vi "FTW-TestExecutive-Core_Process.vi"(0 "FTW Actor Instance Configuration":string="{\n  \"Identity\": \"FTW Test Executive\",\n  \"InboxAddress\": \"inproc://ftwTestExec\",\n  \"LoggerAddress\": \"\",\n  \"Connections\": {},\n  \"Publishers\": {\n    \"TestExecStatus\": \"inproc://testExecStatus\"\n  },\n  \"Subscriptions\": {},\n  \"Step Name Dictionary\": {},\n  \"Refresh Period\": 0.1\n}", 11 "ErrorIn":errorcluster) -> (15 "Error":errorcluster)   [LabVIEW 2015, in "FTW-TestExecutive-Core.lvclass"]
uses:
  FTW-TestExecutive-Core.lvclass
  source/actor/Instance/FTW-ActorInstance.lvclass
  source/actor/Message/Request/FTW-Message-IncomingRequest.lvclass
  source/actor/Message/Base/FTW-Message.lvclass
  source/actor/Instance-Extended/FTW-ActorExtended.lvclass
  Test Steps/Wait/FTW-TestStep-Wait-Core_Step.vi
  Test Steps/Wait/FTW-TestStep-Wait-Core.lvclass
  FTW-TestExecutive-Core_State.ctl
  FTW-TestExecutive-Core_Step_State.ctl
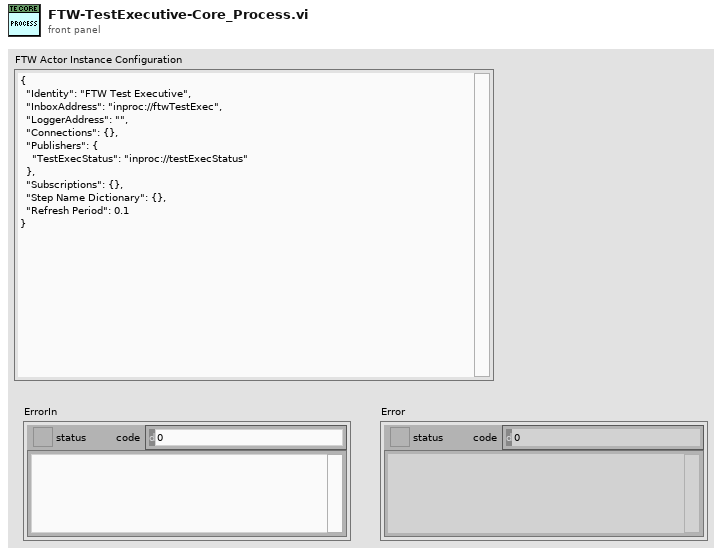
[diagram p1: front panel]
types:
  T1 = cluster{"Incoming Requests":refnum<event-registration>, "Local Messages":refnum<event-registration>, "Subscriber Registration":refnum<event-registration>}
  T2 = typedef "FTW-TestExecutive-Core.lvclass/FTW-TestExecutive-Core_Step_State.ctl" = enum8{"None", "Failed", "Passed", "Timed out", "Aborted"}
  T3 = typedef "FTW-TestExecutive-Core.lvclass/FTW-TestExecutive-Core_State.ctl" = enum8{"Unloaded", "Loaded", "Executing", "Paused"}
  T4 = typedef "FTW-TestExecutive_Step.ctl" = cluster{"Name":string, "Type":string, "Path":string, "Config":string, "Elapsed Time":dbl, "Passed":bool}
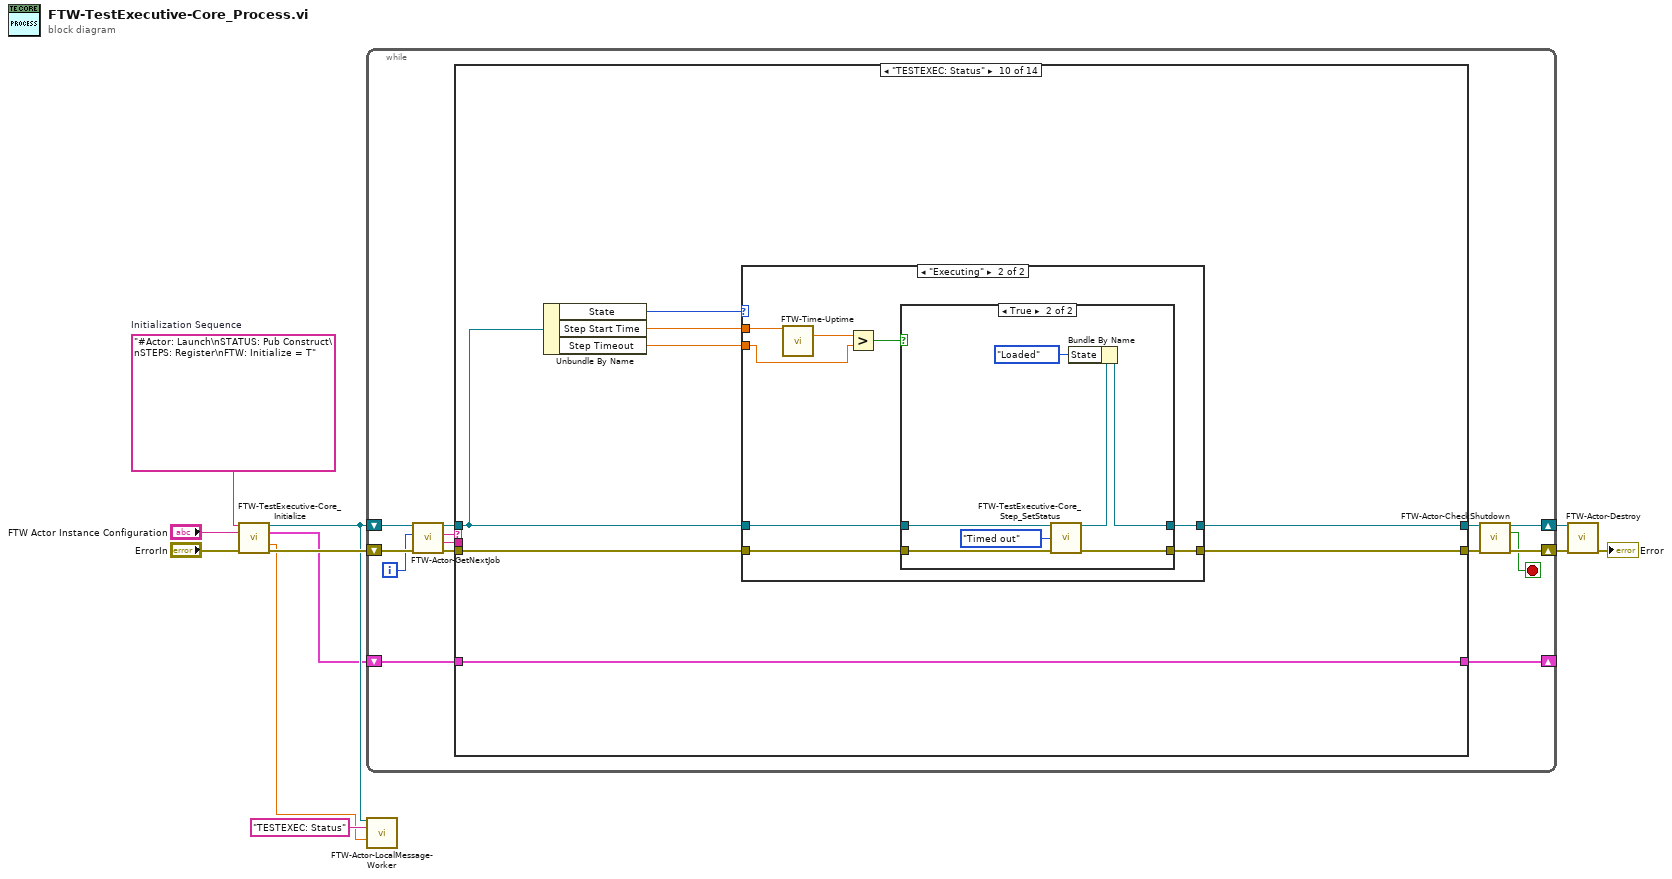
[diagram p0: block diagram]
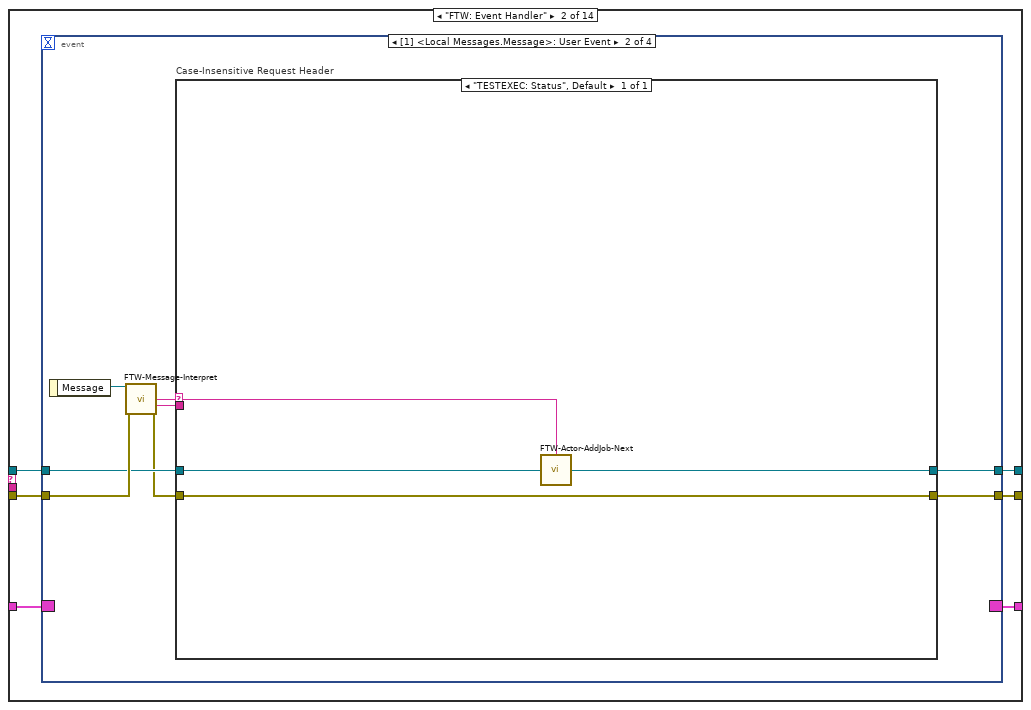
[diagram p3: hidden frame]
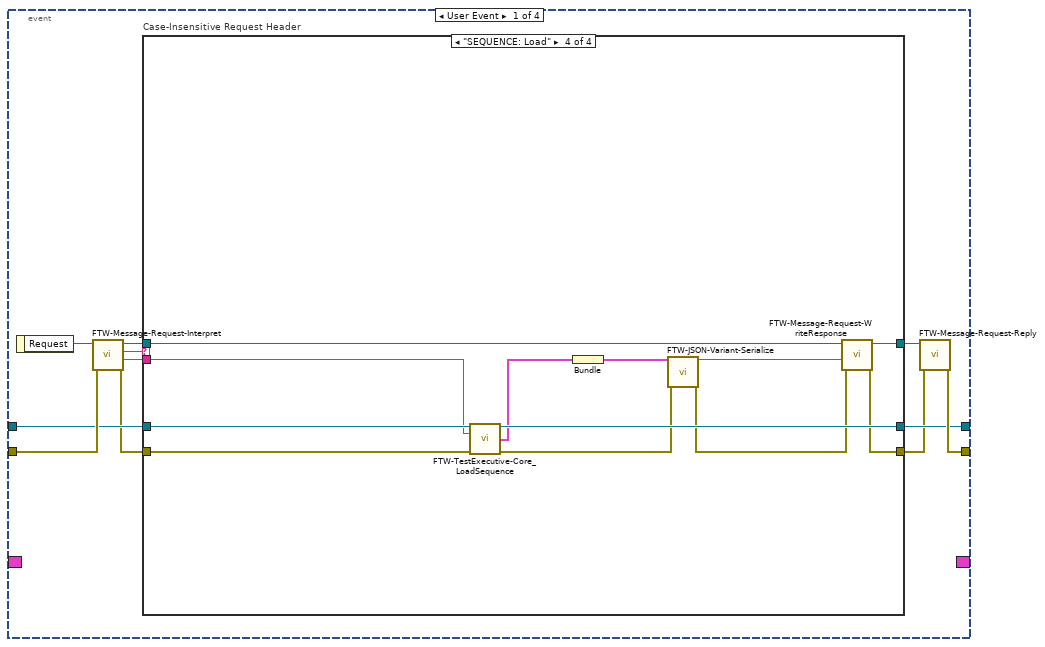
[diagram p4: hidden frame]
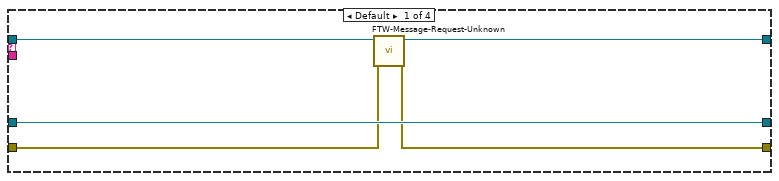
[diagram p5: hidden frame]
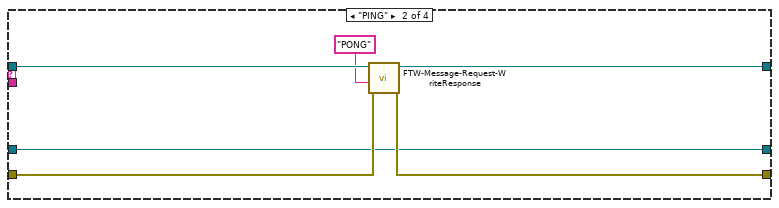
[diagram p6: hidden frame]
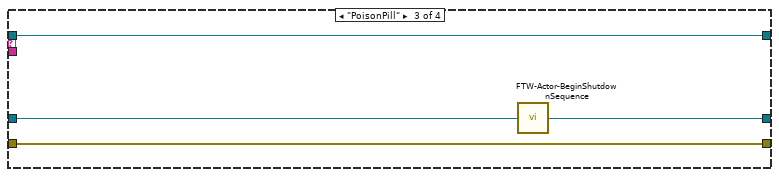
[diagram p7: hidden frame]
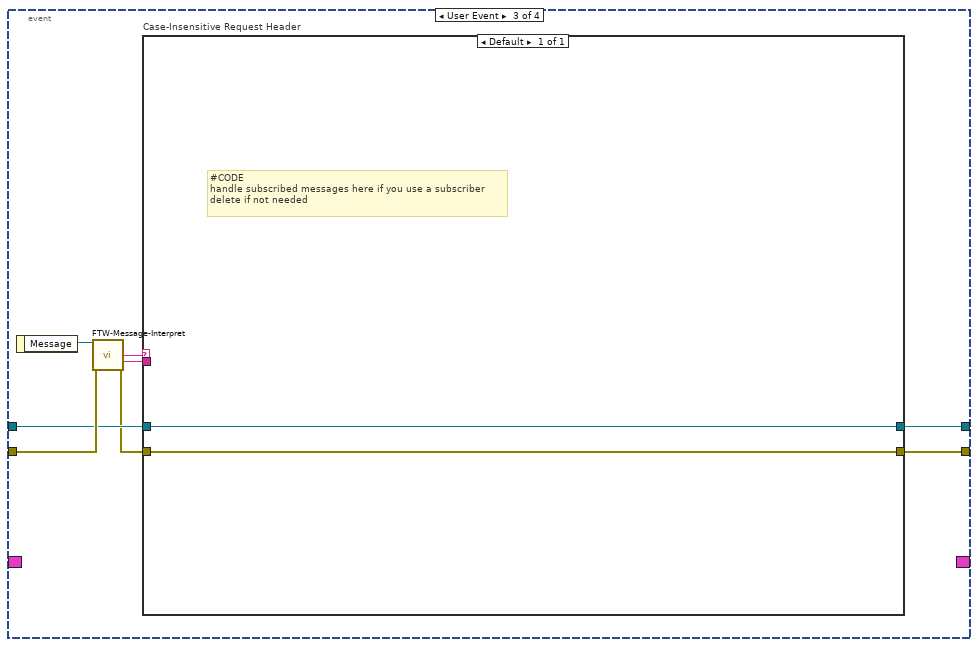
[diagram p8: hidden frame]
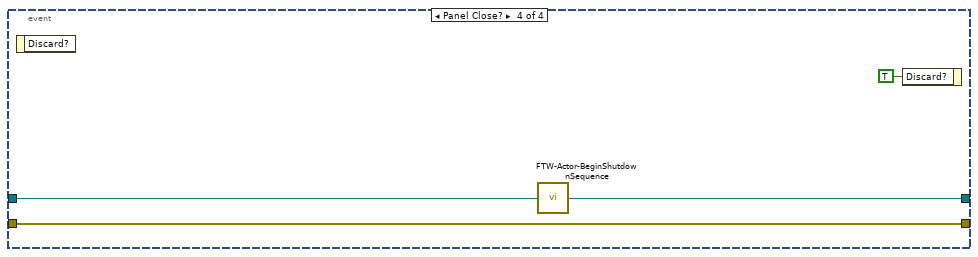
[diagram p9: hidden frame]
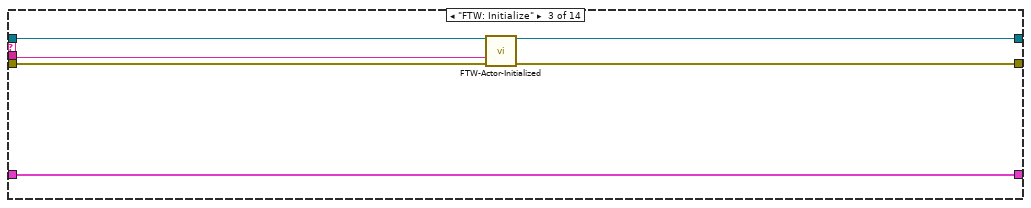
[diagram p10: hidden frame]
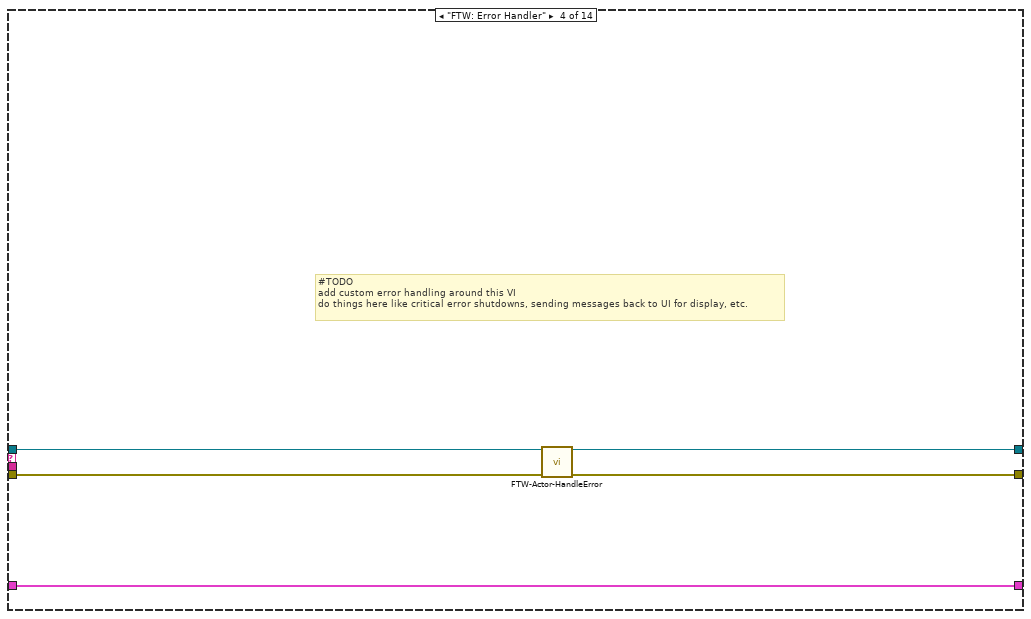
[diagram p11: hidden frame]
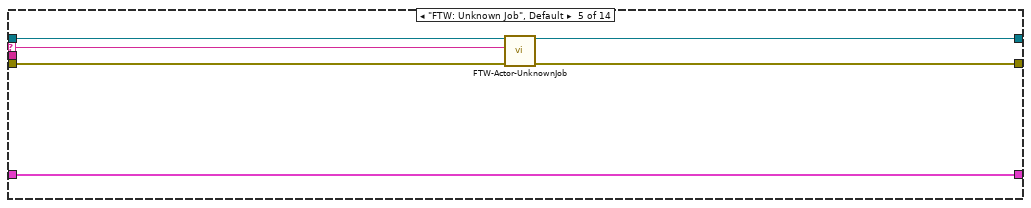
[diagram p12: hidden frame]
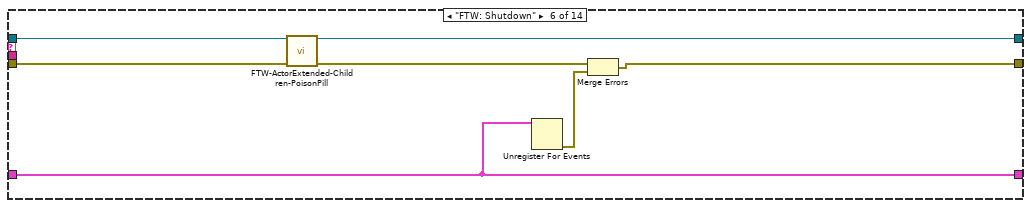
[diagram p13: hidden frame]
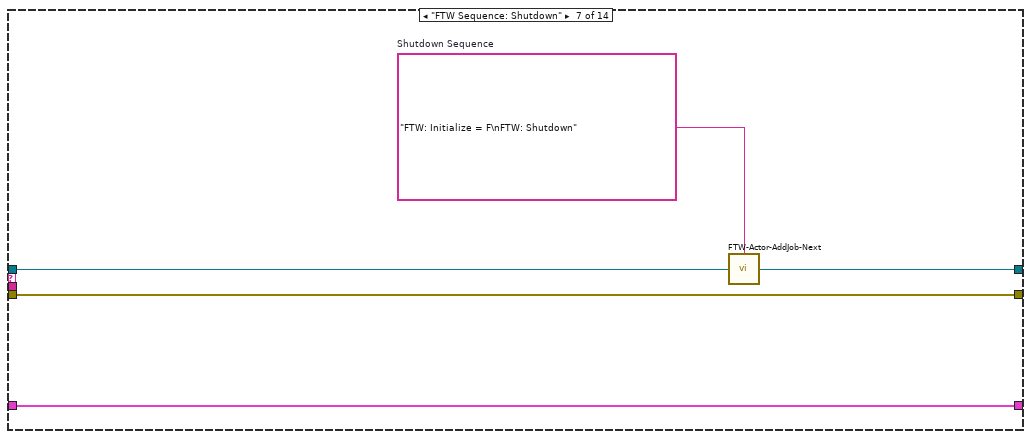
[diagram p14: hidden frame]
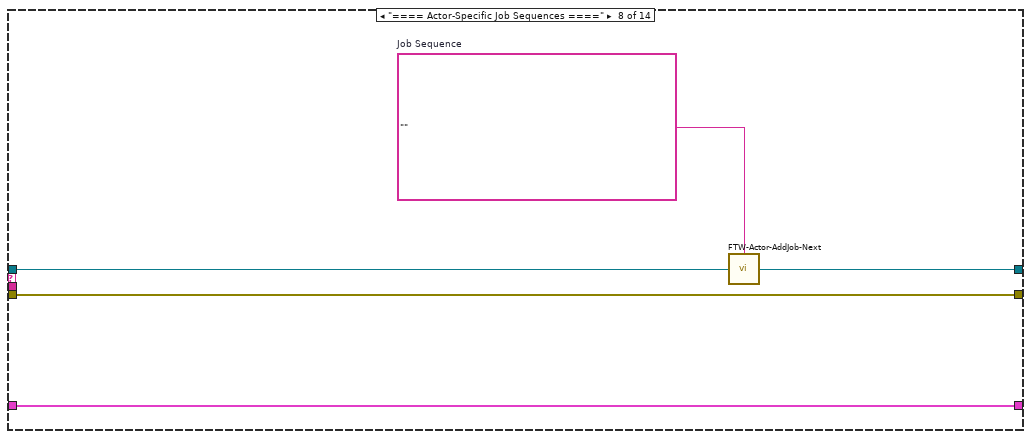
[diagram p15: hidden frame]
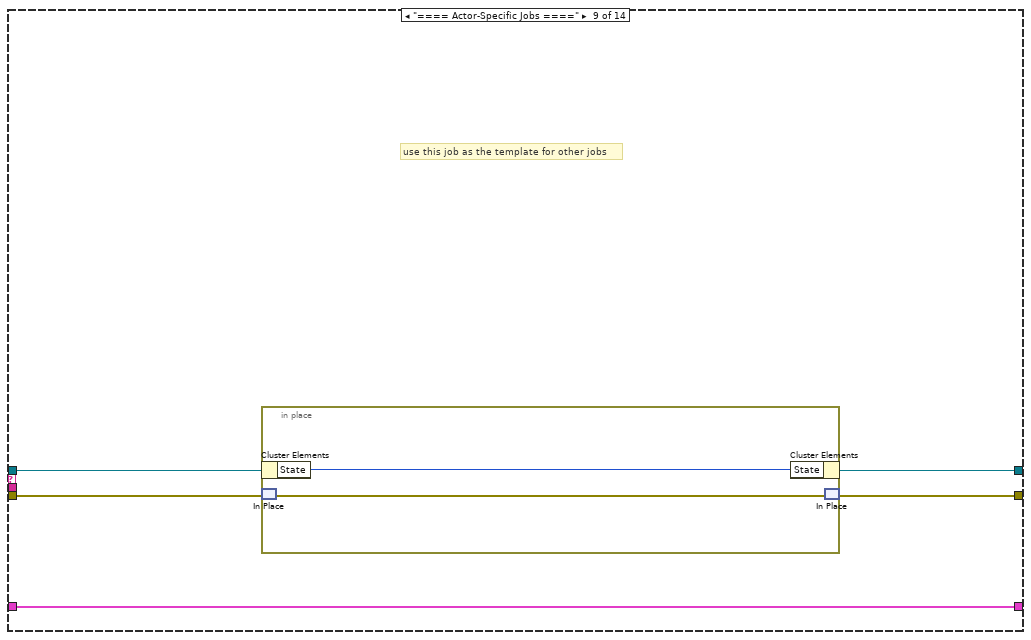
[diagram p16: hidden frame]
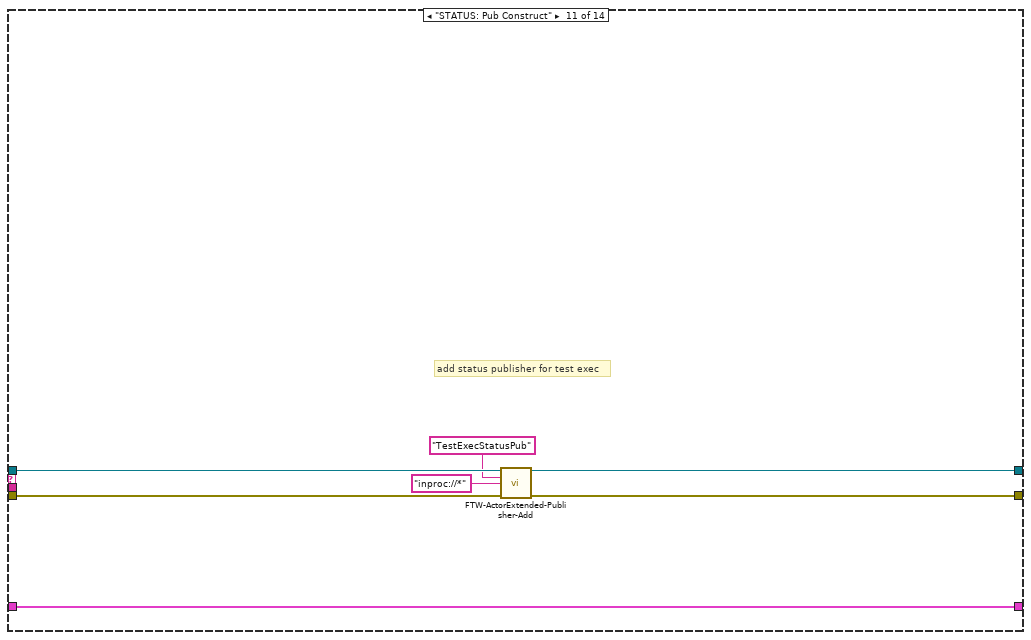
[diagram p19: hidden frame]
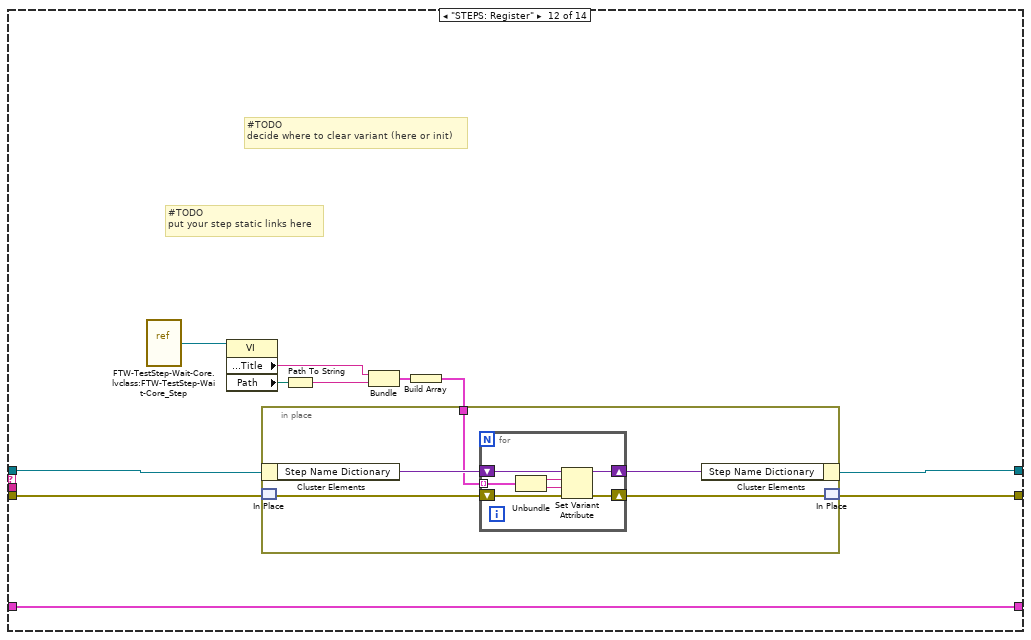
[diagram p20: hidden frame]
diagram:
  w7 = "#Actor: Launch\nSTATUS: Pub Construct\nSTEPS: Register\nFTW: Initialize = T"  # Initialization Sequence
  n1 = call "FTW-TestExecutive-Core_Initialize.vi"("Initialization Sequence"=w7, "FTW Actor Instance Configuration"="FTW Actor Instance Configuration", "error in (no error)"="ErrorIn") -> ("Actor Template-Core out"=w3:refnum<class "FTW-TestExecutive-Core.lvclass">, "Event Refnums"=w1:T1, "Refresh Period"=w2:dbl, "error out"=w8:errorcluster)  [unwired: 9 in]
  n2 = while {
    shift-right: [w15] -> w10
    shift-left: w8 -> [w22]
    shift-right: [w12] -> _
    shift-left: w1 -> [w25]
    shift-right: [w17] -> w11
    shift-left: w3 -> [w24]
    i -> [w13]
    stop <- w14 stop-if-true
    n3 = call "FTW-Actor-GetNextJob.vi"("error in"=w22, "Jobs Performed"=w13, "FTW Actor Instance"=w24) -> ("error out"=w21:errorcluster, "Job Data"=w19:string, "Job Name"=w20:string, "FTW Actor Instance out"=w23:refnum<class "FTW-TestExecutive-Core.lvclass">)  [unwired: 5 in]
    n4 = case shown="\"TESTEXEC: Status\"" w20 {
      selector: w20 -> [_ _ _ _ w110 _ _ _ _ _ _ _ _ _]
      tunnel: [w27 w34 w101 w105 w113 w121 w126 w131 w135 w143 w171 w182 w199 w202] -> w16
      tunnel: w21 -> [w27 w33 w103 w107 w114 w122 w126 w131 w136 w142 w172 w183 w200 w208]
      tunnel: w25 -> [w28 w29 w104 w109 w115 w119 w127 w132 w137 w147 w173 w184 w201 w209]
      tunnel: [w28 w32 w104 w109 w115 w119 w127 w132 w137 w147 w173 w184 w201 w209] -> w12
      tunnel: w19 -> [_ _ w99 _ _ _ _ _ _ _ _ _ _ _]
      tunnel: [w26 w31 w102 w106 w111 w116 w124 w129 w133 w140 w170 w180 w198 w206] -> w18
      tunnel: w23 -> [w26 w30 w100 w108 w112 w117 w125 w130 w134 w141 w169 w181 w197 w207]
      frame "==== Featherweight Framework Jobs ====" {
      }
      frame "FTW: Event Handler" {
        n5 = event shown="[1] <Local Messages.Message>: User Event" {
          selector: w29 -> [_ _ _ _]
          dyn-events: [_ _ _ _] -> w32
          timeout: _ -> [_ _ _ _]
          tunnel: [w44 w75 w87 w97] -> w34
          tunnel: w33 -> [w43 w79 w91 w97]
          tunnel: [w38 w76 w88 w95] -> w31
          tunnel: w30 -> [w42 w78 w90 w96]
          event User Event {
            n6 = event-data() -> ("Request"=w45:refnum<class "FTW-Message-IncomingRequest.lvclass">)  [unwired: 1 in]
            n7 = call "FTW-Message-Request-Interpret.vi"("error in"=w43, "FTW Incoming Request"=w45) -> ("error out"=w41:errorcluster, "Request Body"=w35:string, "Request Header"=w39:string, "FTW Incoming Request out"=w40:refnum<class "FTW-Message-IncomingRequest.lvclass">)  [unwired: 6 in]
            n8 = case "Case-Insensitive Request Header" shown="\"SEQUENCE: Load\"" w39 {
              tunnel: [w48 w54 w59 w63] -> w37
              tunnel: w41 -> [w49 w55 w59 w69]
              tunnel: [w50 w53 w60 w70] -> w38
              tunnel: w42 -> [w50 w53 w58 w71]
              tunnel: w40 -> [w47 w56 w57 w72]
              tunnel: [w46 w52 w57 w67] -> w36
              tunnel: w35 -> [_ _ _ w68]
              frame Default {
                n9 = call "FTW-Message-Request-Unknown.vi"("error in"=w49, "FTW Incoming Request"=w47) -> ("error out"=w48:errorcluster, "FTW Incoming Request Out"=w46:refnum<class "FTW-Message-IncomingRequest.lvclass">)  [unwired: 8 in]
              }
              frame "PING" {
                n10 = call "FTW-Message-Request-WriteResponse.vi"("error in"=w55, "Response Body"="PONG" ("Response Header"), "FTW Incoming Request"=w56) -> ("error out"=w54:errorcluster, "FTW Incoming Request out"=w52:refnum<class "FTW-Message-IncomingRequest.lvclass">)  [unwired: 7 in]
              }
              frame "PoisonPill" {
                n11 = call "FTW-Actor-BeginShutdownSequence.vi"("FTW Actor Instance"=w58) -> ("FTW Actor Instance out"=w60:refnum<class "FTW-TestExecutive-Core.lvclass">)  [unwired: 3 in]
              }
              frame "SEQUENCE: Load" {
                n12 = call "FTW-TestExecutive-Core_LoadSequence.vi"("FTW-Scripter-Core In"=w71, "Sequence"=w68, "error in"=w69) -> ("FTW-Scripter-Core Out"=w70:refnum<class "FTW-TestExecutive-Core.lvclass">, "Loaded Sequence"=w61:T4[], "error out"=w66:errorcluster)  [unwired: 10 in]
                n13 = Bundle("Loaded Sequence"=w61) -> (w62:cluster{"Loaded Sequence":T4[]})  [unwired: 1 in]
                n14 = call "FTW-JSON-Variant-Serialize.vi"("Variant"=w62, "error in"=w66) -> ("JSON String"=w65:string, "error out"=w64:errorcluster)  [unwired: 12 in]
                n15 = call "FTW-Message-Request-WriteResponse.vi"("error in"=w64, "Response Body"=w65, "FTW Incoming Request"=w72) -> ("error out"=w63:errorcluster, "FTW Incoming Request out"=w67:refnum<class "FTW-Message-IncomingRequest.lvclass">)  [unwired: 7 in]
              }
            }
            n16 = call "FTW-Message-Request-Reply.vi"("FTW: Reply Error"=w37, "FTW Incoming Request"=w36) -> ("error out"=w44:errorcluster)  [unwired: 8 in, 1 out]
          }
          event User Event {
            n17 = event-data() -> ("Message"=w80:refnum<class "FTW-Message.lvclass">)  [unwired: 1 in]
            n18 = call-dynamic "FTW-Message-Interpret.vi"("FTW Message"=w80, "error in"=w79) -> ("Message Header"=w74:string, "Message Body"=w73:string, "error out"=w77:errorcluster)  [unwired: 9 in, 2 out]
            n19 = case "Case-Insensitive Request Header" shown="\"TESTEXEC: Status\", Default" w74 {
              selector: w74 -> [w81]
              tunnel: [w83] -> w75
              tunnel: w77 -> [w83]
              tunnel: [w82] -> w76
              tunnel: w78 -> [w84]
              tunnel: w73 -> [_]
              frame "TESTEXEC: Status", Default {
                n20 = call "FTW-Actor-AddJob-Next.vi"("Add Next in Job Queue"=w81, "FTW Actor Instance"=w84) -> ("FTW Actor Instance out"=w82:refnum<class "FTW-TestExecutive-Core.lvclass">)  [unwired: 2 in]
              }
            }
          }
          event User Event {
            n21 = event-data() -> ("Message"=w92:refnum<class "FTW-Message.lvclass">)  [unwired: 1 in]
            n22 = call-dynamic "FTW-Message-Interpret.vi"("FTW Message"=w92, "error in"=w91) -> ("Message Header"=w86:string, "Message Body"=w85:string, "error out"=w89:errorcluster)  [unwired: 9 in, 2 out]
            n23 = case "Case-Insensitive Request Header" shown="Default" w86 {
              tunnel: [w93] -> w87
              tunnel: w89 -> [w93]
              tunnel: [w94] -> w88
              tunnel: w90 -> [w94]
              tunnel: w85 -> [_]
              frame Default {
                # "#CODE\nhandle subscribed messages here if you use a subscriber\ndelete if not needed"
              }
            }
          }
          event Panel Close? {
            n24 = event-data() -> ()  [unwired: 1 in, 1 out]
            n25 = call "FTW-Actor-BeginShutdownSequence.vi"("FTW Actor Instance"=w96) -> ("FTW Actor Instance out"=w95:refnum<class "FTW-TestExecutive-Core.lvclass">)  [unwired: 3 in]
            n26 = event-data("Discard?"=TRUE) -> ()  [unwired: 1 in, 1 out]
          }
        }
      }
      frame "FTW: Initialize" {
        n27 = call-dynamic "FTW-Actor-Initialized.vi"("FTW Actor Instance"=w100, "Positive Init?"=w99, "error in"=w103) -> ("FTW Actor Instance out"=w102:refnum<class "FTW-TestExecutive-Core.lvclass">, "error out"=w101:errorcluster)  [unwired: 11 in]
      }
      frame "FTW: Error Handler" {
        # "#TODO\nadd custom error handling around this VI\ndo things here like critical error shutdowns, sending messages back to UI for display, etc."
        n28 = call-dynamic "FTW-Actor-HandleError.vi"("FTW Actor Instance"=w108, "error in"=w107) -> ("FTW Actor Instance out"=w106:refnum<class "FTW-TestExecutive-Core.lvclass">, "error out"=w105:errorcluster)  [unwired: 10 in, 2 out]
      }
      frame "FTW: Unknown Job", Default {
        n29 = call-dynamic "FTW-Actor-UnknownJob.vi"("FTW Actor Instance"=w112, "Unknown Job"=w110, "error in"=w114) -> ("FTW Actor Instance out"=w111:refnum<class "FTW-TestExecutive-Core.lvclass">, "error out"=w113:errorcluster)  [unwired: 11 in]
      }
      frame "FTW: Shutdown" {
        n30 = call "FTW-ActorExtended-Children-PoisonPill.vi"("FTW-ActorExtended In"=w117, "error in"=w122) -> ("FTW-ActorExtended Out"=w116:refnum<class "FTW-TestExecutive-Core.lvclass">, "error out"=w118:errorcluster)  [unwired: 12 in]
        n31 = Unregister For Events(event registration refnum=w119) -> (error out=w120:errorcluster)  [unwired: 1 in]
        n32 = Merge Errors(w118, w120) -> (w121:errorcluster)
      }
      frame "FTW Sequence: Shutdown" {
        w123 = "FTW: Initialize = F\nFTW: Shutdown"  # Shutdown Sequence
        n33 = call "FTW-Actor-AddJob-Next.vi"("Add Next in Job Queue"=w123, "FTW Actor Instance"=w125) -> ("FTW Actor Instance out"=w124:refnum<class "FTW-TestExecutive-Core.lvclass">)  [unwired: 2 in]
      }
      frame "==== Actor-Specific Job Sequences ====" {
        w128 = ""  # Job Sequence
        n34 = call "FTW-Actor-AddJob-Next.vi"("Add Next in Job Queue"=w128, "FTW Actor Instance"=w130) -> ("FTW Actor Instance out"=w129:refnum<class "FTW-TestExecutive-Core.lvclass">)  [unwired: 2 in]
      }
      frame "==== Actor-Specific Jobs ====" {
        # "use this job as the template for other jobs"
        n35 = in-place {
          n36 = in-place-cluster #1(w134) -> ("State"=w138:T3)
          n37 = in-place-match #2(w136) -> (w139:errorcluster)
          n38 = in-place-cluster #1("State"=w138) -> (w133:refnum<class "FTW-TestExecutive-Core.lvclass">)
          n39 = in-place-match #2(w139) -> (w135:errorcluster)
        }
      }
      frame "TESTEXEC: Status" {
        n40 = Unbundle By Name(w141) -> ("State"=w145:T3, "Step Start Time"=w146:dbl, "Step Timeout"=w144:dbl)
        n41 = case shown="\"Executing\"" w145 {
          tunnel: w146 -> [_ w157]
          tunnel: w144 -> [_ w155]
          tunnel: [w148 w152] -> w143
          tunnel: w142 -> [w148 w154]
          tunnel: w141 -> [w149 w151]
          tunnel: [w149 w153] -> w140
          frame "Unloaded", "Loaded" {
          }
          frame "Executing" {
            n42 = call "FTW-Time-Uptime.vi"("Previous Uptime"=w157) -> ("Elapsed Time"=w156:dbl)  [unwired: 12 in, 2 out]
            n43 = Greater?(x=w156, y=w155) -> (0:w150:bool)
            n44 = case shown="True" w150 {
              tunnel: w154 -> [w158 w166]
              tunnel: [w159 w165] -> w153
              tunnel: [w158 w163] -> w152
              tunnel: w151 -> [w159 w162]
              frame False {
              }
              frame True {
                n45 = call "FTW-TestExecutive-Core_Step_SetStatus.vi"("FTW-Scripter-Core In"=w162, "State"=FTW-TestExecutive-Core_Step_State."Timed out", "error in"=w166) -> ("FTW-Scripter-Core Out"=w161:refnum<class "FTW-TestExecutive-Core.lvclass">, "error out"=w163:errorcluster)  [unwired: 11 in]
                n46 = Bundle By Name(cluster=w161, "State"=FTW-TestExecutive-Core_State."Loaded") -> (w165:refnum<class "FTW-TestExecutive-Core.lvclass">)
              }
            }
          }
        }
      }
      frame "STATUS: Pub Construct" {
        # "add status publisher for test exec"
        n47 = call "FTW-ActorExtended-Publisher-Add.vi"("FTW-ActorExtended In"=w169, "Publisher Name"="TestExecStatusPub", "Publisher URI"="inproc://*", "error in"=w172) -> ("FTW-ActorExtended Out"=w170:refnum<class "FTW-TestExecutive-Core.lvclass">, "error out"=w171:errorcluster)  [unwired: 10 in]
      }
      frame "STEPS: Register" {
        # "#TODO\nput your step static links here"
        # "#TODO\ndecide where to clear variant (here or init)"
        n48 = vi-ref "FTW-TestStep-Wait-Core.lvclass:FTW-TestStep-Wait-Core_Step.vi"() -> (w179:refnum<vi>)
        n49 = property class="VI"(reference=w179) -> ("Front Panel.Title"=w175:string, "Path"=w178:path)  [unwired: 1 in, 2 out]
        n50 = Path To String(path=w178) -> (string=w177:string)
        n51 = Bundle("Front Panel.Title"=w175, w177) -> (w176:cluster{"Front Panel.Title":string, string})  [unwired: 1 in]
        n52 = Build Array(w176) -> (w174:cluster{"Front Panel.Title":string, string}[])
        n53 = in-place {
          in-place-border: w174 -> [w185]
          n54 = in-place-cluster #3(w181) -> ("Step Name Dictionary"=w187:variant)
          n55 = in-place-match #4(w183) -> (w189:errorcluster)
          n56 = for {
            shift-right: [w195] -> w188
            shift-left: w189 -> [w196]
            shift-right: [w193] -> w186
            shift-left: w187 -> [w194]
            tunnel: w185 -> [w192] mode=indexing
            n57 = Unbundle(w192) -> ("Front Panel.Title"=w191:string, w190:string)
            n58 = Set Variant Attribute(Variant=w194, name=w191, value=w190, error in=w196) -> (Variant out=w193:variant, error out=w195:errorcluster)  [unwired: 1 out]
          }
          n59 = in-place-cluster #3("Step Name Dictionary"=w186) -> (w180:refnum<class "FTW-TestExecutive-Core.lvclass">)
          n60 = in-place-match #4(w188) -> (w182:errorcluster)
        }
      }
      frame "STEP: Execute" {
        n61 = call "FTW-TestExecutive-Core_Step_Launch.vi"("FTW-Scripter-Core In"=w197, "error in"=w200) -> ("FTW-Scripter-Core Out"=w198:refnum<class "FTW-TestExecutive-Core.lvclass">, "error out"=w199:errorcluster)  [unwired: 12 in]
      }
      frame "CONN: Ask" {
        # "example of asking a connected actor something\n\nuse the connection to call the actor API"
        n62 = call "FTW-ActorExtended-Connection-Get.vi"("FTW-ActorExtended In"=w207, "Connector Name"="ConnectionOne" ("Publisher Name"), "error in"=w208) -> ("FTW-ActorExtended Out"=w206:refnum<class "FTW-TestExecutive-Core.lvclass">, "FTW Actor Connector"=w204:refnum<class "FTW-ActorConnector.lvclass">, "error out"=w203:errorcluster)  [unwired: 10 in]
        n63 = flat-sequence {
          tunnel: w204 -> [_]
          tunnel: w203 -> [w210]
          tunnel: [w210] -> w202
          frame #0 {
          }
        }
      }
    }
    n64 = call "FTW-Actor-CheckShutdown.vi"("FTW Actor Instance"=w18, "error in"=w16) -> ("FTW Actor Instance out"=w17:refnum<class "FTW-TestExecutive-Core.lvclass">, "Shutdown?"=w14:bool, "error out"=w15:errorcluster)  [unwired: 11 in]
  }
  n65 = call-dynamic "FTW-Actor-LocalMessage-Worker.vi"("FTW-ActorInstance In"=w3, "Message Header"="TESTEXEC: Status", "Send Rate"=w2) -> ()  [unwired: 13 in]
  n66 = call-dynamic "FTW-Actor-Destroy.vi"("FTW Actor Instance"=w11, "error in"=w10) -> ("error out"=→"Error":errorcluster)  [unwired: 13 in]
